vi "Ann_int.vi"(0 "Data":dbl[](array[numeric]), 1 "Loss Function":enum16{"MSE", "MAE"}(ring), 2 "Regularization":T1, 5 "Target":dbl format="%#_13g", 7 "Training?":bool, 9 "Parameters":T3, 13 "Adam Data In":T2) -> (4 "Output":dbl, 6 "Error":dbl, 10 "Adjusted Parameters":T3, 14 "Adam Data Out":T2, 15 "Data Output":dbl)   [LabVIEW 2020]
uses:
  Sub-VIs/Adam_data.ctl
  Sub-VIs/Globals.vi
  Sub-VIs/Layer.vi
  Sub-VIs/Layer1d.vi
panel:
  out "Error Codes":i32[](array[numeric])
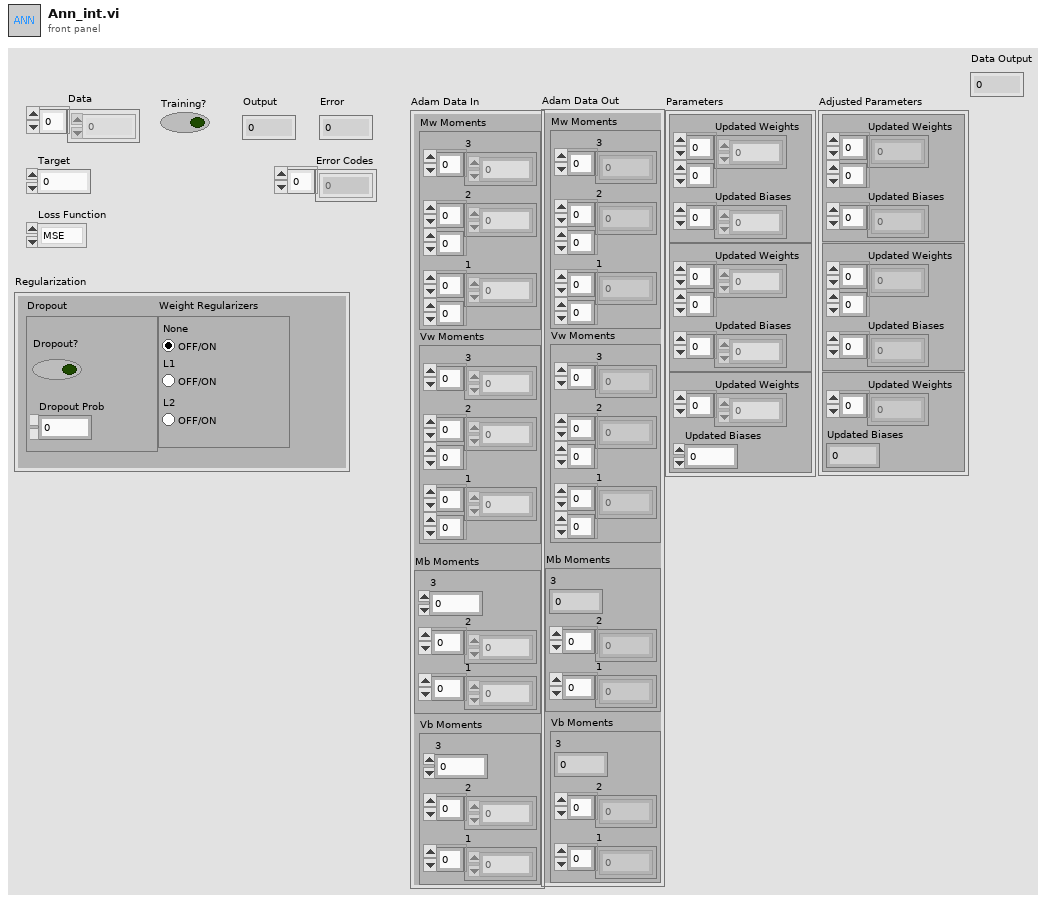
[diagram p1: front panel]
types:
  T1 = cluster{"Dropout":cluster{"Dropout?":bool, "Dropout Prob":dbl}, "Weight Regularizers":enum32{"None", "L1", "L2"}}
  T2 = typedef "Adam_data.ctl" = cluster{"Mw Moments":cluster{"3 ":dbl[], "2":dbl[][], "1":dbl[][]}, "Vw Moments":cluster{"3":dbl[], "2":dbl[][], "1":dbl[][]}, "Mb Moments":cluster{"3":dbl, "2":dbl[], "1":dbl[]}, "Vb Moments":cluster{"3":dbl, "2":dbl[], "1":dbl[]}}
  T3 = cluster{cluster{"Updated Weights":dbl[][], "Updated Biases":dbl[]}, cluster{"Updated Weights":dbl[][], "Updated Biases":dbl[]}, cluster{"Updated Weights":dbl[], "Updated Biases":dbl}}
  T4 = cluster{"Updated Weights":dbl[][], "Updated Biases":dbl[]}
  T5 = cluster{"Updated Weights":dbl[], "Updated Biases":dbl}
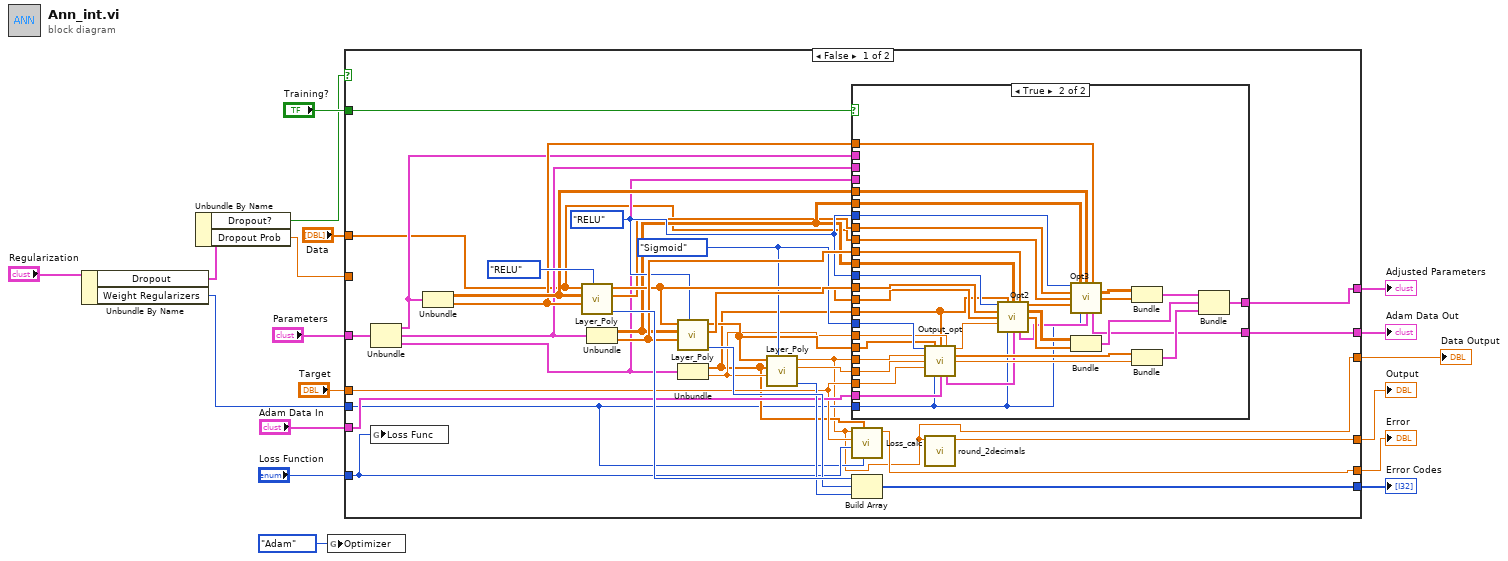
[diagram p0: block diagram]
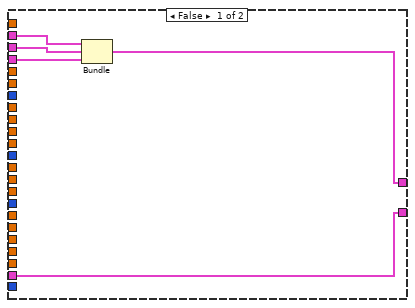
[diagram p2: hidden frame]
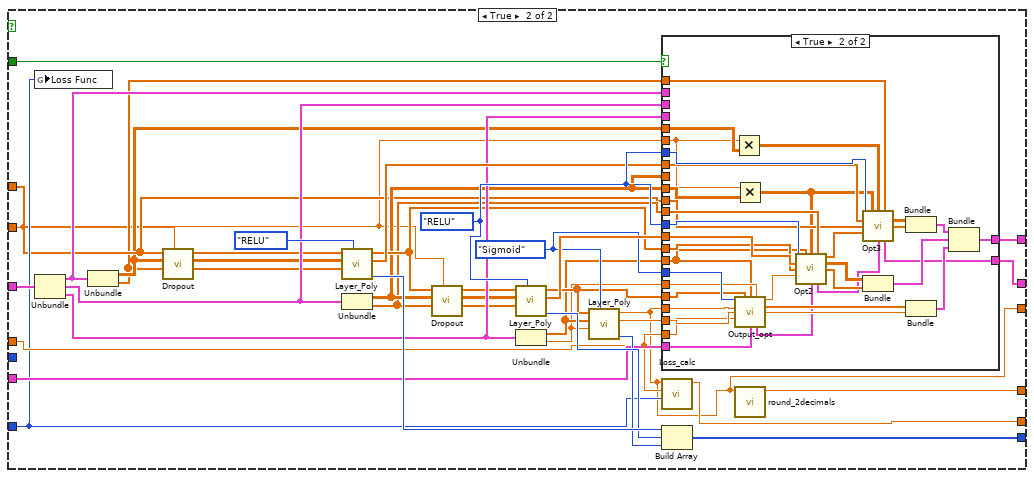
[diagram p3: hidden frame]
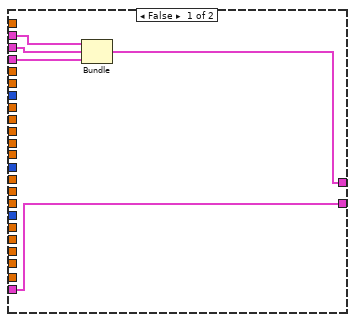
[diagram p4: hidden frame]
diagram:
  n1 = Unbundle By Name("Regularization") -> ("Dropout"=w5:cluster{"Dropout?":bool, "Dropout Prob":dbl}, "Weight Regularizers"=w2:enum32{"None", "L1", "L2"})
  n2 = Unbundle By Name(w5) -> ("Dropout?"=w4:bool, "Dropout Prob"=w3:dbl)
  n3 = global write "Globals.vi" "Optimizer"(enum16{"Adagrad", "Adadelta", "Adam"}."Adam" ("Optimizer")) -> ()
  n4 = case shown="False" w4 {
    tunnel: "Parameters" -> [w32 w115]
    tunnel: "Data" -> [w31 w99]
    tunnel: "Training?" -> [w30 w114]
    tunnel: "Adam Data In" -> [w29 w113]
    tunnel: [w28 w112] -> w13
    tunnel: [w27 w111] -> w12
    tunnel: "Target" -> [w26 w110]
    tunnel: [w25 w109] -> w10
    tunnel: [w24 w108] -> w9
    tunnel: "Loss Function" -> [w23 w107]
    tunnel: [w22 w106] -> w7
    tunnel: w3 -> [_ w93]
    tunnel: w2 -> [w20 _]
    tunnel: [w19 w92] -> w1
    frame False {
      w39 = enum32{"Sigmoid", "RELU", "Tanh", "Leaky RELU"}."Sigmoid" ("Activation Function")
      w44 = enum32{"Sigmoid", "RELU", "Tanh", "Leaky RELU"}."RELU" ("Activation Function")
      n5 = Unbundle(w32) -> (w36:T4, w35:T4, w34:T5)
      n6 = global write "Globals.vi" "Loss Func"(w23) -> ()
      n7 = Unbundle(w36) -> ("Updated Weights"=w42:dbl[][], "Updated Biases"=w41:dbl[])
      n8 = call-poly "Layer_Poly.vi"("Activation Function"=enum32{"Sigmoid", "RELU", "Tanh", "Leaky RELU"}."RELU", "Biases"=w41, "Weights"=w42, "Data"=w31) -> ("Error"=w51:i32, "Net Activation"=w40:dbl[], "Output"=w45:dbl[])  [unwired: 5 in]
      n9 = Unbundle(w35) -> ("Updated Weights"=w43:dbl[][], "Updated Biases"=w47:dbl[])
      n10 = call-poly "Layer_Poly.vi"("Activation Function"=w44, "Biases"=w47, "Weights"=w43, "Data"=w45) -> ("Error"=w50:i32, "Net Activation"=w46:dbl[], "Output"=w38:dbl[])  [unwired: 5 in]
      n11 = Unbundle(w34) -> ("Updated Weights"=w21:dbl[], "Updated Biases"=w33:dbl)
      n12 = call-poly "Layer_Poly.vi"("Activation Function"=w39, "Biases"=w33, "Weights"=w21, "Data"=w38) -> ("Error"=w49:i32, "Net Activation"=w37:dbl, "Output"=w19:dbl)  [unwired: 5 in]
      n13 = case shown="True" w30 {
        tunnel: w44 -> [_ w91]
        tunnel: w43 -> [_ w90]
        tunnel: w47 -> [_ w89]
        tunnel: w46 -> [_ w88]
        tunnel: w45 -> [_ w87]
        tunnel: w44 -> [_ w86]
        tunnel: w43 -> [_ w85]
        tunnel: w42 -> [_ w84]
        tunnel: w41 -> [_ w83]
        tunnel: w40 -> [_ w82]
        tunnel: w31 -> [_ w81]
        tunnel: w39 -> [_ w79]
        tunnel: w38 -> [_ w78]
        tunnel: w19 -> [_ w77]
        tunnel: w37 -> [_ w76]
        tunnel: w26 -> [_ w75]
        tunnel: [w53 w60] -> w28
        tunnel: w36 -> [w56 _]
        tunnel: w35 -> [w55 _]
        tunnel: w34 -> [w54 _]
        tunnel: w21 -> [_ w67]
        tunnel: w33 -> [_ w68]
        tunnel: [w52 w59] -> w27
        tunnel: w29 -> [w52 w58]
        tunnel: w20 -> [_ w57]
        frame False {
          n14 = Bundle(w56, w55, w54) -> (w53:T3)  [unwired: 1 in]
        }
        frame True {
          n15 = call "Output_opt.vi"("Activation Function"=w79, "Activation l-1"=w78, "Weights"=w67, "Biases"=w68, "Activation"=w77, "Net Output"=w76, "Target"=w75, "Weight Regularizers"=w57, "Adam Data In"=w58) -> ("Delta"=w74:dbl, "Updated Weights"=w71:dbl[], "Updated Biases"=w70:dbl, "Adam Data Out"=w62:T2)  [unwired: 3 in]
          n16 = call "Opt2.vi"("Activation Function"=w91, "Weights l+1"=w67, "Weights"=w90, "Biases"=w89, "Net Output"=w88, "Activations l-1"=w87, "Delta l+1"=w74, "Weight Regularizers"=w57, "Adam Data In"=w62) -> ("Delta l"=w80:dbl[], "Updated Weights"=w66:dbl[][], "Updated Biases"=w65:dbl[], "Adam Data Out"=w61:T2)  [unwired: 3 in]
          n17 = call "Opt3.vi"("Activation Function"=w86, "Weights l+1"=w85, "Weights"=w84, "Biases"=w83, "Net Output"=w82, "Activations l-1"=w81, "Delta l+1"=w80, "Weight Regularizers"=w57, "Adam Data In"=w61) -> ("Updated Weights"=w64:dbl[][], "Updated Biases"=w63:dbl[], "Adam Data Out"=w59:T2)  [unwired: 4 in]
          n18 = Bundle("Updated Weights"=w66, "Updated Biases"=w65) -> (w73:T4)  [unwired: 1 in]
          n19 = Bundle("Updated Weights"=w64, "Updated Biases"=w63) -> (w72:T4)  [unwired: 1 in]
          n20 = Bundle("Updated Weights"=w71, "Updated Biases"=w70) -> (w69:T5)  [unwired: 1 in]
          n21 = Bundle(w72, w73, w69) -> (w60:T3)  [unwired: 1 in]
        }
      }
      n22 = call "Loss_calc.vi"("Weight Regularizers"=w20, "Weights"=w21, "Loss Type"=w23, "Target"=w26, "Data"=w19) -> ("Loss"=w25:dbl)  [unwired: 6 in]
      n23 = Build Array(w51, w50, w49) -> (w24:i32[])
      n24 = call "round_2decimals.vi"("Number"=w19) -> ("Rounded Number"=w22:dbl)  [unwired: 10 in]
    }
    frame True {
      w123 = enum32{"Sigmoid", "RELU", "Tanh", "Leaky RELU"}."Sigmoid" ("Activation Function")
      w125 = enum32{"Sigmoid", "RELU", "Tanh", "Leaky RELU"}."RELU" ("Activation Function")
      n25 = global write "Globals.vi" "Loss Func"(w107) -> ()
      n26 = Unbundle(w115) -> (w120:T4, w119:T4, w118:T5)
      n27 = Unbundle(w120) -> ("Updated Weights"=w98:dbl[][], "Updated Biases"=w97:dbl[])
      n28 = call "Dropout.vi"("Droput Prob"=w93, "Biases"=w97, "Weights"=w98, "Data"=w99) -> ("Droupout Biases"=w94:dbl[], "Dropout Weights"=w95:dbl[][], "Droput Data"=w96:dbl[])  [unwired: 5 in]
      n29 = call-poly "Layer_Poly.vi"("Activation Function"=enum32{"Sigmoid", "RELU", "Tanh", "Leaky RELU"}."RELU", "Biases"=w94, "Weights"=w95, "Data"=w96) -> ("Error"=w130:i32, "Net Activation"=w124:dbl[], "Output"=w105:dbl[])  [unwired: 5 in]
      n30 = Unbundle(w119) -> ("Updated Weights"=w104:dbl[][], "Updated Biases"=w103:dbl[])
      n31 = call "Dropout.vi"("Droput Prob"=w93, "Biases"=w103, "Weights"=w104, "Data"=w105) -> ("Droupout Biases"=w100:dbl[], "Dropout Weights"=w101:dbl[][], "Droput Data"=w102:dbl[])  [unwired: 5 in]
      n32 = call-poly "Layer_Poly.vi"("Activation Function"=w125, "Biases"=w100, "Weights"=w101, "Data"=w102) -> ("Error"=w129:i32, "Net Activation"=w126:dbl[], "Output"=w122:dbl[])  [unwired: 5 in]
      n33 = Unbundle(w118) -> ("Updated Weights"=w117:dbl[], "Updated Biases"=w116:dbl)
      n34 = call-poly "Layer_Poly.vi"("Activation Function"=w123, "Biases"=w116, "Weights"=w117, "Data"=w122) -> ("Error"=w128:i32, "Net Activation"=w121:dbl, "Output"=w92:dbl)  [unwired: 5 in]
      n35 = case shown="True" w114 {
        tunnel: w125 -> [_ w171]
        tunnel: w104 -> [_ w140]
        tunnel: w103 -> [_ w170]
        tunnel: w126 -> [_ w169]
        tunnel: w105 -> [_ w168]
        tunnel: w125 -> [_ w167]
        tunnel: w104 -> [_ _]
        tunnel: w98 -> [_ w138]
        tunnel: w97 -> [_ w166]
        tunnel: w124 -> [_ w165]
        tunnel: w99 -> [_ w164]
        tunnel: w123 -> [_ w162]
        tunnel: w122 -> [_ w161]
        tunnel: w92 -> [_ w160]
        tunnel: w121 -> [_ w159]
        tunnel: w110 -> [_ w158]
        tunnel: [w132 w143] -> w112
        tunnel: w120 -> [w135 _]
        tunnel: w119 -> [w134 _]
        tunnel: w118 -> [w133 _]
        tunnel: w117 -> [_ w150]
        tunnel: w116 -> [_ w151]
        tunnel: [w131 w142] -> w111
        tunnel: w113 -> [w131 w141]
        tunnel: w93 -> [_ w136]
        frame False {
          n36 = Bundle(w135, w134, w133) -> (w132:T3)  [unwired: 1 in]
        }
        frame True {
          n37 = Multiply(x=w136, y=w138) -> (x*y=w137:dbl[][])
          n38 = Multiply(x=w136, y=w140) -> (x*y=w139:dbl[][])
          n39 = call "Output_opt.vi"("Activation Function"=w162, "Activation l-1"=w161, "Weights"=w150, "Biases"=w151, "Activation"=w160, "Net Output"=w159, "Target"=w158, "Adam Data In"=w141) -> ("Delta"=w157:dbl, "Updated Weights"=w154:dbl[], "Updated Biases"=w153:dbl, "Adam Data Out"=w145:T2)  [unwired: 4 in]
          n40 = call "Opt2.vi"("Activation Function"=w171, "Weights l+1"=w150, "Weights"=w139, "Biases"=w170, "Net Output"=w169, "Activations l-1"=w168, "Delta l+1"=w157, "Adam Data In"=w145) -> ("Delta l"=w163:dbl[], "Updated Weights"=w149:dbl[][], "Updated Biases"=w148:dbl[], "Adam Data Out"=w144:T2)  [unwired: 4 in]
          n41 = call "Opt3.vi"("Activation Function"=w167, "Weights l+1"=w139, "Weights"=w137, "Biases"=w166, "Net Output"=w165, "Activations l-1"=w164, "Delta l+1"=w163, "Adam Data In"=w144) -> ("Updated Weights"=w147:dbl[][], "Updated Biases"=w146:dbl[], "Adam Data Out"=w142:T2)  [unwired: 5 in]
          n42 = Bundle("Updated Weights"=w149, "Updated Biases"=w148) -> (w156:T4)  [unwired: 1 in]
          n43 = Bundle("Updated Weights"=w147, "Updated Biases"=w146) -> (w155:T4)  [unwired: 1 in]
          n44 = Bundle("Updated Weights"=w154, "Updated Biases"=w153) -> (w152:T5)  [unwired: 1 in]
          n45 = Bundle(w155, w156, w152) -> (w143:T3)  [unwired: 1 in]
        }
      }
      n46 = call "Loss_calc.vi"("Loss Type"=w107, "Target"=w110, "Data"=w92) -> ("Loss"=w109:dbl)  [unwired: 8 in]
      n47 = Build Array(w130, w129, w128) -> (w108:i32[])
      n48 = call "round_2decimals.vi"("Number"=w92) -> ("Rounded Number"=w106:dbl)  [unwired: 10 in]
    }
  }
  "Adjusted Parameters" <- w13
  "Adam Data Out" <- w12
  "Error" <- w10
  "Error Codes" <- w9
  "Output" <- w7
  "Data Output" <- w1
